vi "forloop.vi"() -> ()   [LabVIEW 2015]
panel:
  out "?":string
  out "?":dbl
  out "?":string
  out "?":dbl
  in  "number":dbl
  out "Numeric":i32
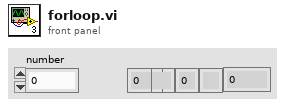
[diagram p1: front panel]
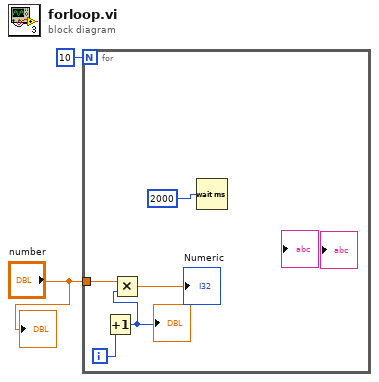
[diagram p0: block diagram]
diagram:
  n1 = for {
    N: 10 -> [_]
    tunnel: "number" -> [w6]
    i -> [w4]
    n2 = Increment(x=w4) -> (x+1=w3:i32)
    "?" <- w3
    n3 = Multiply(x=w6, y=w3) -> (x*y=→"Numeric":dbl)
    n4 = Wait (ms)(milliseconds to wait=u32 2000) -> ()  [unwired: 1 out]
  }
  "?" <- "number"
